vi "SENS_CORR_COLL_GUID_ADAP_DESC.vi"(0 "VISA IN":refnum<visa-resource-name>, 1 "Adapter Index":i32, 2 "Desc":string, 5 "error in":errorcluster, 7 "Channel":i32=1) -> (14 "VISA Out":refnum<visa-resource-name>, 19 "error out":errorcluster)   [LabVIEW 2018, in "PNA-X.lvlib"]
doc: "SENSe<cnum>:CORRection:COLLect:GUIDed:ADAPter<n>:DESCription <string> \n1644\n\n(Write-only) Specifies the adapter description for use as the guided cal connection prompts. \nParameters \n<cnum> Any existing channel number. If unspecified, value is set to 1 \n<n> Adapter index number that was returned from \nSENS:CORR:COLL:GUID:ADAP:CREate? \n<string> Adapter description. \nExamples See example using this command. \nQuery Syntax Not Applicable \nDefault Not Applicable"
uses:
  PNA-X.lvlib
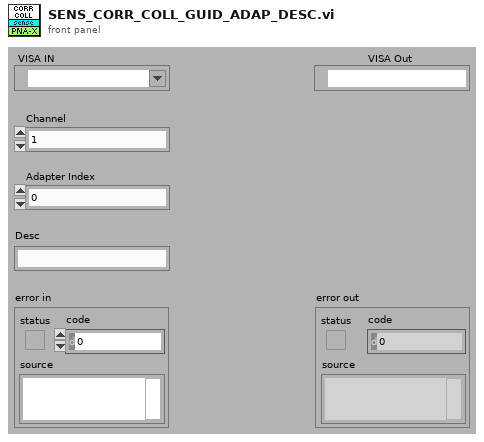
[diagram p1: front panel]
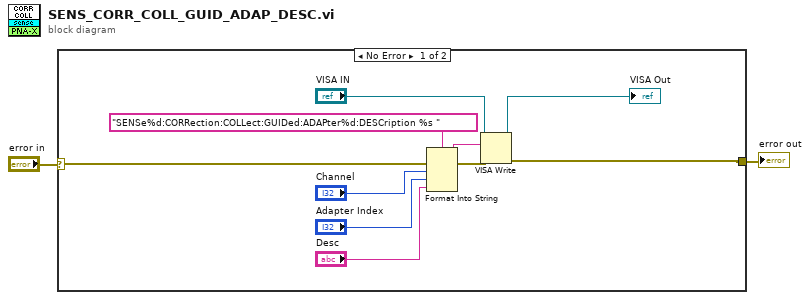
[diagram p0: block diagram]
diagram:
  n1 = case shown="No Error" "error in" {
    selector: "error in" -> [w12 w13]
    tunnel: [w7 w13] -> w1
    frame No Error {
      n2 = Format Into String(format string="SENSe%d:CORRection:COLLect:GUIDed:ADAPter%d:DESCription %s " ("Cmdline"), error in=w12, "Channel", "Adapter Index", "Desc") -> (resulting string=w10:string, error out=w11:errorcluster)  [unwired: 1 in]
      n3 = VISA Write(VISA resource name="VISA IN", write buffer=w10, error in (no error)=w11) -> (VISA resource name out=→"VISA Out":refnum<visa-resource-name>, error out=w7:errorcluster)  [unwired: 1 out]
    }
    frame Error {
    }
  }
  "error out" <- w1
